vi "Water Tank.vi"() -> ()   [LabVIEW 2013]
uses:
  Water Tank Global.vi
panel:
  in  "Stop Fill":bool
  in  "Start Fill":bool
  out "Bottom Float Switch":bool
  out "Top Float Switch":bool
  out "Water level":i32(slide) scale=0.0..300.0
  # "Click          to run"
  # "Water Tank"
  # "Here, there is a 300 gallon water tank that drains at a constant rate of 50 gal/sec. There is a water pump that adds water at a rate of 100 gal/sec.\n\nYour job is to add this functionality:\nThe water pump is activated by the Start Fill button. When this starts, water gets pumped into the tank until it hits the top float switch. Once this switch is tripped, the water pump turns off.  \nThe water level keeps decreasing until it the water level goes below the bottom float switch. At this point, the water pump should start back up and restart the cycle. The water level should oscillate between the two levels like this until the stop fill button is pushed, at which point the tank will drain."
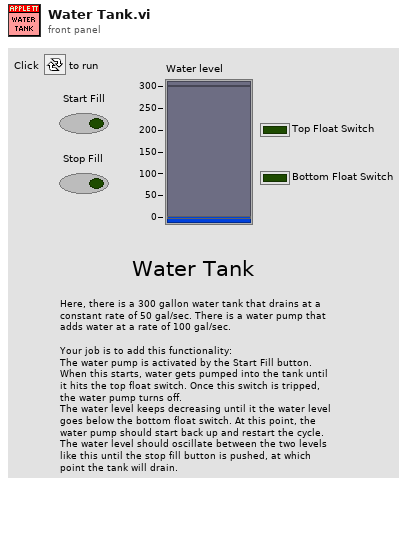
[diagram p1: front panel]
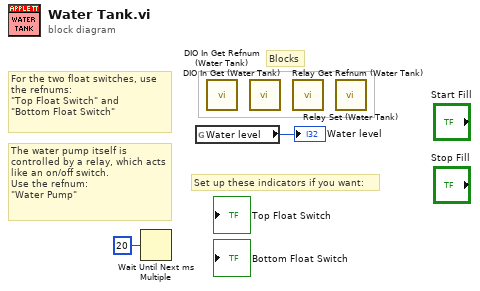
[diagram p0: block diagram]
diagram:
  # "The water pump itself is controlled by a relay, which acts like an on/off switch.\nUse the refnum:\n\"Water Pump\""
  # "For the two float switches, use\nthe refnums:\n\"Top Float Switch\" and\n\"Bottom Float Switch\""
  # "Set up these indicators if you want:"
  # "Blocks"
  n1 = Wait Until Next ms Multiple(millisecond multiple=u32 20) -> ()  [unwired: 1 out]
  n2 = global read "Water Tank Global.vi" "Water level"() -> (→"Water level":i32)
  n3 = call "DIO In Get Refnum (Water Tank).vi"() -> ()  [unwired: 10 in, 2 out]
  n4 = call "DIO In Get (Water Tank).vi"() -> ()  [unwired: 9 in, 3 out]
  n5 = call "Relay Get Refnum (Water Tank).vi"() -> ()  [unwired: 10 in, 2 out]
  n6 = call "Relay Set (Water Tank).vi"() -> ()  [unwired: 10 in, 2 out]
